vi "Test Set Active.vi"(8 "error in (no error)":errorcluster) -> (0 "error out":errorcluster)   [LabVIEW 2019]
uses:
  <vilib>/addons/_JKI Toolkits/Caraya/classes/Test/Test.lvclass
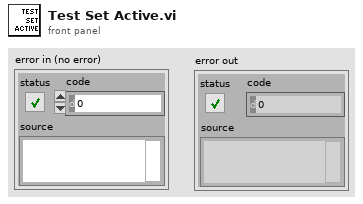
[diagram p1: front panel]
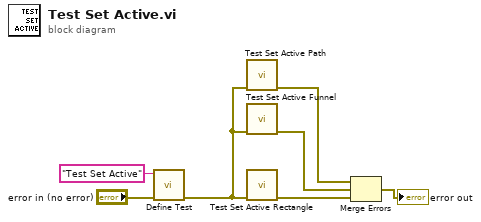
[diagram p0: block diagram]
diagram:
  n1 = call <vilib>:"Define Test.vi"("error in (no error)"="error in (no error)", "Label (VI Title)"="Test Set Active") -> ("error out"=w2:errorcluster)  [unwired: 8 in, 1 out]
  n2 = call "Test Set Active Path.vi"("error in (no error)"=w2) -> ("error out"=w1:errorcluster)  [unwired: 10 in]
  n3 = call "Test Set Active Funnel.vi"("error in (no error)"=w2) -> ("error out"=w3:errorcluster)  [unwired: 10 in]
  n4 = call "Test Set Active Rectangle.vi"("error in (no error)"=w2) -> ("error out"=w4:errorcluster)  [unwired: 10 in]
  n5 = Merge Errors(w1, w3, w4) -> (→"error out":errorcluster)
